vi "VI Tree.vi"   [LabVIEW 2017, in "Keithley 2600 Series.lvlib"]
doc: "This is the instrument driver for the Keithley 2600 Series. The VI Tree displays all the user-callable VIs of the instrument driver in an organized table."
uses:
  <instrlib>/Keithley 2600 Series/Keithley 2600 Series.lvlib
  <instrlib>/Keithley 2600 Series/Public/Data/Read Current (Linear Voltage Sweep).vi
  <instrlib>/Keithley 2600 Series/Public/Data/Read Voltage (Linear Current Sweep).vi
  <instrlib>/Keithley 2600 Series/Public/Configure/Factory Script/Configure Tag Current Pulse (Linear).vi
  <instrlib>/Keithley 2600 Series/Public/Configure/Factory Script/Configure Tag Voltage Pulse (Linear).vi
  <instrlib>/Keithley 2600 Series/Public/Configure/Source/Configure Source (Level).vi
  <instrlib>/Keithley 2600 Series/Public/Data/Read Asynchronous Measurement (Current).vi
  <instrlib>/Keithley 2600 Series/Public/Data/Read Measurement (Current).vi
  <instrlib>/Keithley 2600 Series/Public/Data/Read Transconductance (Current).vi
panel:
  # "(c) 2019 National Instruments.  ALL RIGHTS RESERVED."
  # "SEE DIAGRAM\nFOR VI TREE."
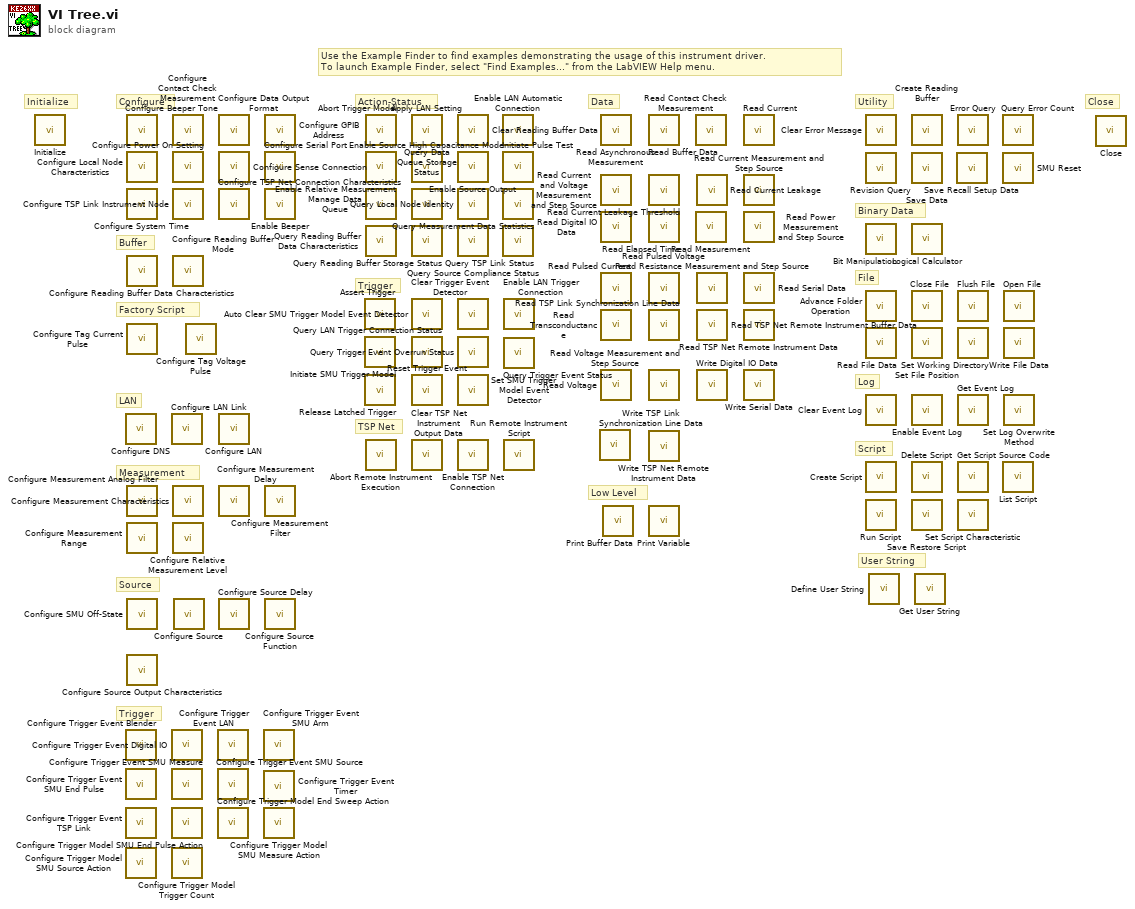
[diagram p0: block diagram]
diagram:
  # "Close"
  # "User String"
  # "Script"
  # "Log"
  # "File"
  # "Binary Data"
  # "Utility"
  # "Low Level"
  # "Data"
  # "Trigger"
  # "Source"
  # "Measurement"
  # "LAN"
  # "Factory Script"
  # "Buffer"
  # "Configure"
  # "TSP Net"
  # "Trigger"
  # "Action-Status"
  # "Initialize"
  # "Use the Example Finder to find examples demonstrating the usage of this instrument driver.\nTo launch Example Finder, select \"Find Examples...\" from the LabVIEW Help menu."
  n1 = call <instrlib>:"Initialize.vi"() -> ()  [unwired: 10 in, 2 out]
  n2 = call <instrlib>:"Configure DNS.vi"() -> ()  [unwired: 14 in, 2 out]
  n3 = call <instrlib>:"Configure Trigger Event Blender.vi"() -> ()  [unwired: 14 in, 2 out]
  n4 = call <instrlib>:"Configure Trigger Event SMU End Pulse.vi"() -> ()  [unwired: 14 in, 2 out]
  n5 = call <instrlib>:"Configure Trigger Event TSP Link.vi"() -> ()  [unwired: 14 in, 2 out]
  n6 = call <instrlib>:"Configure Trigger Model SMU Source Action.vi"() -> ()  [unwired: 18 in, 2 out]
  n7 = call <instrlib>:"Configure Beeper Tone.vi"() -> ()  [unwired: 10 in, 2 out]
  n8 = call <instrlib>:"Configure Local Node Characteristics.vi"() -> ()  [unwired: 14 in, 2 out]
  n9 = call <instrlib>:"Configure System Time.vi"() -> ()  [unwired: 10 in, 2 out]
  n10 = call <instrlib>:"Configure Reading Buffer Data Characteristics.vi"() -> ()  [unwired: 10 in, 2 out]
  n11 = call-poly <instrlib>:"Configure Tag Current Pulse.vi"() -> ()  [unwired: 26 in, 2 out]
  n12 = call <instrlib>:"Configure Measurement Analog Filter.vi"() -> ()  [unwired: 10 in, 2 out]
  n13 = call <instrlib>:"Configure Measurement Range.vi"() -> ()  [unwired: 14 in, 2 out]
  n14 = call <instrlib>:"Configure SMU Off-State.vi"() -> ()  [unwired: 10 in, 2 out]
  n15 = call <instrlib>:"Configure Source Output Characteristics.vi"() -> ()  [unwired: 10 in, 2 out]
  n16 = call <instrlib>:"Configure LAN Link.vi"() -> ()  [unwired: 14 in, 2 out]
  n17 = call <instrlib>:"Configure Trigger Event Digital IO.vi"() -> ()  [unwired: 14 in, 2 out]
  n18 = call <instrlib>:"Configure Trigger Event SMU Measure.vi"() -> ()  [unwired: 14 in, 2 out]
  n19 = call <instrlib>:"Configure Trigger Model SMU End Pulse Action.vi"() -> ()  [unwired: 14 in, 2 out]
  n20 = call <instrlib>:"Configure Trigger Model Trigger Count.vi"() -> ()  [unwired: 10 in, 2 out]
  n21 = call <instrlib>:"Configure Contact Check Measurement.vi"() -> ()  [unwired: 10 in, 2 out]
  n22 = call <instrlib>:"Configure Power On Setting.vi"() -> ()  [unwired: 10 in, 2 out]
  n23 = call <instrlib>:"Configure TSP Link Instrument Node.vi"() -> ()  [unwired: 10 in, 2 out]
  n24 = call <instrlib>:"Configure Reading Buffer Mode.vi"() -> ()  [unwired: 14 in, 2 out]
  n25 = call <instrlib>:"Configure Measurement Characteristics.vi"() -> ()  [unwired: 10 in, 2 out]
  n26 = call <instrlib>:"Configure Relative Measurement Level.vi"() -> ()  [unwired: 14 in, 2 out]
  n27 = call-poly <instrlib>:"Configure Source.vi"() -> ()  [unwired: 14 in, 2 out]
  n28 = call-poly <instrlib>:"Configure Tag Voltage Pulse.vi"() -> ()  [unwired: 26 in, 2 out]
  n29 = call <instrlib>:"Configure Trigger Event LAN.vi"() -> ()  [unwired: 14 in, 2 out]
  n30 = call <instrlib>:"Configure Trigger Event SMU Source.vi"() -> ()  [unwired: 14 in, 2 out]
  n31 = call <instrlib>:"Configure Trigger Model End Sweep Action.vi"() -> ()  [unwired: 10 in, 2 out]
  n32 = call <instrlib>:"Configure Data Output Format.vi"() -> ()  [unwired: 10 in, 2 out]
  n33 = call <instrlib>:"Configure Sense Connection.vi"() -> ()  [unwired: 10 in, 2 out]
  n34 = call <instrlib>:"Configure TSP Net Connection Characteristics.vi"() -> ()  [unwired: 10 in, 2 out]
  n35 = call <instrlib>:"Configure LAN.vi"() -> ()  [unwired: 10 in, 2 out]
  n36 = call <instrlib>:"Configure Measurement Delay.vi"() -> ()  [unwired: 10 in, 2 out]
  n37 = call <instrlib>:"Configure Source Delay.vi"() -> ()  [unwired: 10 in, 2 out]
  n38 = call <instrlib>:"Configure Trigger Event SMU Arm.vi"() -> ()  [unwired: 14 in, 2 out]
  n39 = call <instrlib>:"Configure Trigger Event Timer.vi"() -> ()  [unwired: 14 in, 2 out]
  n40 = call <instrlib>:"Configure Trigger Model SMU Measure Action.vi"() -> ()  [unwired: 14 in, 2 out]
  n41 = call <instrlib>:"Configure GPIB Address.vi"() -> ()  [unwired: 10 in, 2 out]
  n42 = call <instrlib>:"Configure Serial Port.vi"() -> ()  [unwired: 10 in, 2 out]
  n43 = call <instrlib>:"Enable Beeper.vi"() -> ()  [unwired: 10 in, 2 out]
  n44 = call <instrlib>:"Configure Measurement Filter.vi"() -> ()  [unwired: 10 in, 2 out]
  n45 = call <instrlib>:"Configure Source Function.vi"() -> ()  [unwired: 10 in, 2 out]
  n46 = call <instrlib>:"Assert Trigger.vi"() -> ()  [unwired: 10 in, 2 out]
  n47 = call <instrlib>:"Initiate SMU Trigger Model.vi"() -> ()  [unwired: 10 in, 2 out]
  n48 = call <instrlib>:"Release Latched Trigger.vi"() -> ()  [unwired: 10 in, 2 out]
  n49 = call <instrlib>:"Abort Trigger Model.vi"() -> ()  [unwired: 10 in, 2 out]
  n50 = call <instrlib>:"Enable Relative Measurement.vi"() -> ()  [unwired: 10 in, 2 out]
  n51 = call <instrlib>:"Manage Data Queue.vi"() -> ()  [unwired: 9 in, 3 out]
  n52 = call <instrlib>:"Query Reading Buffer Data Characteristics.vi"() -> ()  [unwired: 9 in, 7 out]
  n53 = call <instrlib>:"Abort Remote Instrument Execution.vi"() -> ()  [unwired: 10 in, 2 out]
  n54 = call <instrlib>:"Apply LAN Setting.vi"() -> ()  [unwired: 10 in, 2 out]
  n55 = call <instrlib>:"Enable Source High Capacitance Mode.vi"() -> ()  [unwired: 10 in, 2 out]
  n56 = call <instrlib>:"Query Data Queue Storage Status.vi"() -> ()  [unwired: 8 in, 4 out]
  n57 = call <instrlib>:"Query Reading Buffer Storage Status.vi"() -> ()  [unwired: 7 in, 5 out]
  n58 = call <instrlib>:"Auto Clear SMU Trigger Model Event Detector.vi"() -> ()  [unwired: 10 in, 2 out]
  n59 = call <instrlib>:"Query LAN Trigger Connection Status.vi"() -> ()  [unwired: 9 in, 3 out]
  n60 = call <instrlib>:"Reset Trigger Event.vi"() -> ()  [unwired: 10 in, 2 out]
  n61 = call <instrlib>:"Clear TSP Net Instrument Output Data.vi"() -> ()  [unwired: 10 in, 2 out]
  n62 = call <instrlib>:"Clear Reading Buffer Data.vi"() -> ()  [unwired: 10 in, 2 out]
  n63 = call <instrlib>:"Enable Source Output.vi"() -> ()  [unwired: 10 in, 2 out]
  n64 = call <instrlib>:"Query Local Node Identity.vi"() -> ()  [unwired: 7 in, 5 out]
  n65 = call <instrlib>:"Query Source Compliance Status.vi"() -> ()  [unwired: 9 in, 3 out]
  n66 = call <instrlib>:"Clear Trigger Event Detector.vi"() -> ()  [unwired: 10 in, 2 out]
  n67 = call <instrlib>:"Query Trigger Event Overrun Status.vi"() -> ()  [unwired: 9 in, 3 out]
  n68 = call <instrlib>:"Set SMU Trigger Model Event Detector.vi"() -> ()  [unwired: 10 in, 2 out]
  n69 = call <instrlib>:"Enable TSP Net Connection.vi"() -> ()  [unwired: 14 in, 2 out]
  n70 = call <instrlib>:"Enable LAN Automatic Connection.vi"() -> ()  [unwired: 10 in, 2 out]
  n71 = call <instrlib>:"Initiate Pulse Test.vi"() -> ()  [unwired: 10 in, 2 out]
  n72 = call <instrlib>:"Query Measurement Data Statistics.vi"() -> ()  [unwired: 9 in, 3 out]
  n73 = call <instrlib>:"Query TSP Link Status.vi"() -> ()  [unwired: 9 in, 3 out]
  n74 = call <instrlib>:"Enable LAN Trigger Connection.vi"() -> ()  [unwired: 10 in, 2 out]
  n75 = call <instrlib>:"Query Trigger Event Status.vi"() -> ()  [unwired: 9 in, 3 out]
  n76 = call <instrlib>:"Run Remote Instrument Script.vi"() -> ()  [unwired: 10 in, 2 out]
  n77 = call <instrlib>:"Write TSP Link Synchronization Line Data.vi"() -> ()  [unwired: 10 in, 2 out]
  n78 = call-poly <instrlib>:"Read Asynchronous Measurement.vi"() -> ()  [unwired: 9 in, 3 out]
  n79 = call <instrlib>:"Read Current and Voltage Measurement and Step Source.vi"() -> ()  [unwired: 8 in, 4 out]
  n80 = call <instrlib>:"Read Digital IO Data.vi"() -> ()  [unwired: 8 in, 4 out]
  n81 = call <instrlib>:"Read Pulsed Current.vi"() -> ()  [unwired: 13 in, 3 out]
  n82 = call-poly <instrlib>:"Read Transconductance.vi"() -> ()  [unwired: 11 in, 5 out]
  n83 = call-poly <instrlib>:"Read Voltage.vi"() -> ()  [unwired: 9 in, 3 out]
  n84 = call <instrlib>:"Print Buffer Data.vi"() -> ()  [unwired: 9 in, 3 out]
  n85 = call <instrlib>:"Read Buffer Data.vi"() -> ()  [unwired: 7 in, 5 out]
  n86 = call <instrlib>:"Read Current Leakage Threshold.vi"() -> ()  [unwired: 13 in, 3 out]
  n87 = call <instrlib>:"Read Elapsed Time.vi"() -> ()  [unwired: 9 in, 3 out]
  n88 = call <instrlib>:"Read Pulsed Voltage.vi"() -> ()  [unwired: 13 in, 3 out]
  n89 = call <instrlib>:"Read TSP Link Synchronization Line Data.vi"() -> ()  [unwired: 8 in, 4 out]
  n90 = call <instrlib>:"Read Voltage Measurement and Step Source.vi"() -> ()  [unwired: 9 in, 3 out]
  n91 = call <instrlib>:"Write TSP Net Remote Instrument Data.vi"() -> ()  [unwired: 10 in, 2 out]
  n92 = call <instrlib>:"Print Variable.vi"() -> ()  [unwired: 8 in, 4 out]
  n93 = call <instrlib>:"Read Contact Check Measurement.vi"() -> ()  [unwired: 7 in, 5 out]
  n94 = call-poly <instrlib>:"Read Measurement.vi"() -> ()  [unwired: 8 in, 4 out]
  n95 = call <instrlib>:"Read Current Leakage.vi"() -> ()  [unwired: 13 in, 3 out]
  n96 = call <instrlib>:"Read Resistance Measurement and Step Source.vi"() -> ()  [unwired: 9 in, 3 out]
  n97 = call <instrlib>:"Read TSP Net Remote Instrument Buffer Data.vi"() -> ()  [unwired: 9 in, 3 out]
  n98 = call <instrlib>:"Write Digital IO Data.vi"() -> ()  [unwired: 10 in, 2 out]
  n99 = call-poly <instrlib>:"Read Current.vi"() -> ()  [unwired: 9 in, 3 out]
  n100 = call <instrlib>:"Read Current Measurement and Step Source.vi"() -> ()  [unwired: 9 in, 3 out]
  n101 = call <instrlib>:"Read Power Measurement and Step Source.vi"() -> ()  [unwired: 9 in, 3 out]
  n102 = call <instrlib>:"Read Serial Data.vi"() -> ()  [unwired: 9 in, 3 out]
  n103 = call <instrlib>:"Read TSP Net Remote Instrument Data.vi"() -> ()  [unwired: 9 in, 3 out]
  n104 = call <instrlib>:"Write Serial Data.vi"() -> ()  [unwired: 10 in, 2 out]
  n105 = call <instrlib>:"Clear Error Message.vi"() -> ()  [unwired: 10 in, 2 out]
  n106 = call <instrlib>:"Revision Query.vi"() -> ()  [unwired: 8 in, 4 out]
  n107 = call <instrlib>:"Bit Manipulation.vi"() -> ()  [unwired: 9 in, 3 out]
  n108 = call <instrlib>:"Advance Folder Operation.vi"() -> ()  [unwired: 10 in, 6 out]
  n109 = call <instrlib>:"Read File Data.vi"() -> ()  [unwired: 9 in, 3 out]
  n110 = call <instrlib>:"Clear Event Log.vi"() -> ()  [unwired: 10 in, 2 out]
  n111 = call <instrlib>:"Create Script.vi"() -> ()  [unwired: 10 in, 2 out]
  n112 = call <instrlib>:"Run Script.vi"() -> ()  [unwired: 10 in, 2 out]
  n113 = call <instrlib>:"Define User String.vi"() -> ()  [unwired: 10 in, 2 out]
  n114 = call <instrlib>:"Create Reading Buffer.vi"() -> ()  [unwired: 10 in, 2 out]
  n115 = call <instrlib>:"Save Data.vi"() -> ()  [unwired: 14 in, 2 out]
  n116 = call <instrlib>:"Logical Calculator.vi"() -> ()  [unwired: 9 in, 3 out]
  n117 = call <instrlib>:"Close File.vi"() -> ()  [unwired: 10 in, 2 out]
  n118 = call <instrlib>:"Set File Position.vi"() -> ()  [unwired: 8 in, 4 out]
  n119 = call <instrlib>:"Enable Event Log.vi"() -> ()  [unwired: 10 in, 2 out]
  n120 = call <instrlib>:"Delete Script.vi"() -> ()  [unwired: 10 in, 2 out]
  n121 = call <instrlib>:"Save Restore Script.vi"() -> ()  [unwired: 10 in, 2 out]
  n122 = call <instrlib>:"Get User String.vi"() -> ()  [unwired: 9 in, 3 out]
  n123 = call <instrlib>:"Save Recall Setup Data.vi"() -> ()  [unwired: 10 in, 2 out]
  n124 = call <instrlib>:"Error Query.vi"() -> ()  [unwired: 8 in, 4 out]
  n125 = call <instrlib>:"Flush File.vi"() -> ()  [unwired: 10 in, 2 out]
  n126 = call <instrlib>:"Set Working Directory.vi"() -> ()  [unwired: 9 in, 3 out]
  n127 = call <instrlib>:"Get Event Log.vi"() -> ()  [unwired: 8 in, 4 out]
  n128 = call <instrlib>:"Get Script Source Code.vi"() -> ()  [unwired: 9 in, 3 out]
  n129 = call <instrlib>:"Set Script Characteristic.vi"() -> ()  [unwired: 10 in, 2 out]
  n130 = call <instrlib>:"Query Error Count.vi"() -> ()  [unwired: 9 in, 3 out]
  n131 = call <instrlib>:"SMU Reset.vi"() -> ()  [unwired: 10 in, 2 out]
  n132 = call <instrlib>:"List Script.vi"() -> ()  [unwired: 9 in, 3 out]
  n133 = call <instrlib>:"Open File.vi"() -> ()  [unwired: 10 in, 2 out]
  n134 = call <instrlib>:"Write File Data.vi"() -> ()  [unwired: 10 in, 2 out]
  n135 = call <instrlib>:"Set Log Overwrite Method.vi"() -> ()  [unwired: 10 in, 2 out]
  n136 = call <instrlib>:"Close.vi"() -> ()  [unwired: 11 in, 1 out]
